vi "WPI_SonarSRF04DigitalGetRange.vi"(8 "error in (no error)":errorcluster, 10 "Range Units":T1, 11 "UltrasonicDevRef":T2={"DevStatus"={"status"=FALSE, "code"=0, "source"=""}, "Ping Channel"=enum."Invalid", "Echo Channel"=enum."Invalid", "CntIndex"=enum."Invalid"}) -> (0 "error out":errorcluster, 2 "Distance":dbl, 3 "UltrasonicDevRef":T2={"DevStatus"={"status"=FALSE, "code"=0, "source"=""}, "Ping Channel"=enum."Invalid", "Echo Channel"=enum."Invalid", "CntIndex"=enum."Invalid"})   [LabVIEW 2017]
doc: "Returns the distance, in inches or millimeters, between the ultrasonic sensor and the closest object in front of the sensor. The ultrasonic sensor measures this distance by emitting a ping and calculating the time it takes for the echo of the ping to return. If the ultrasonic sensor does not detect the echo of the ping in 50 ms or less, the VI times out and returns a <B>Distance</B> value of 0.\n\nThis software is licensed. Open the labview\\readme\\WPI Robotics Library Open Source License.txt file for more information."
uses:
  <vilib>/Rock Robotics/WPI/Ultrasonic/WPI_UltrasonicDeviceRef.ctl
  <vilib>/Rock Robotics/SystemInterfaces/DIO/FPGA_DIOChannel.ctl
  <vilib>/Rock Robotics/SystemInterfaces/Counter/FPGA_CounterCtrSystemIndex.ctl
  <vilib>/Rock Robotics/WPI/Ultrasonic/WPI_UltrasonicRangeUnits.ctl
  <instrlib>/Devantech SRF05/HAIOL/Devantech SRF05.lvclass
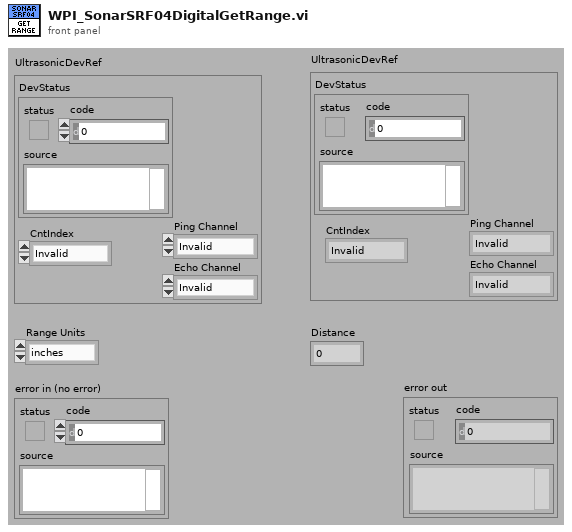
[diagram p1: front panel]
types:
  T1 = typedef "WPI_UltrasonicRangeUnits.ctl" = enum16{"inches", "mm"}
  T2 = typedef "WPI_UltrasonicDeviceRef.ctl" = cluster{"DevStatus":errorcluster, "Ping Channel":T3, "Echo Channel":T3, "CntIndex":T4}
  T3 = typedef "FPGA_DIOChannel.ctl" = enum8{"DIO 0", "DIO 1", "DIO 2", "DIO 3", "DIO 4", "DIO 5", "DIO 6", "DIO 7", "DIO 8", "DIO 9", "DIO MXP 0", "DIO MXP 1", "DIO MXP 2", "DIO MXP 3", "DIO MXP 4", "DIO MXP 5", "DIO MXP 6", "DIO MXP 7", "DIO MXP 8", "DIO MXP 9", "DIO MXP 10", "DIO MXP 11", "DIO MXP 12", "DIO MXP 13", "DIO MXP 14", "DIO MXP 15", "SPI Port CS1", "SPI Port CS2", "SPI Port CS3", "SPI Port MISO", "SPI Port MOSI", "Invalid"}
  T4 = typedef "FPGA_CounterCtrSystemIndex.ctl" = enum8{"Ctr 0", "Ctr 1", "Ctr 2", "Ctr 3", "Ctr 4", "Ctr 5", "Ctr 6", "Ctr 7", "Invalid"}
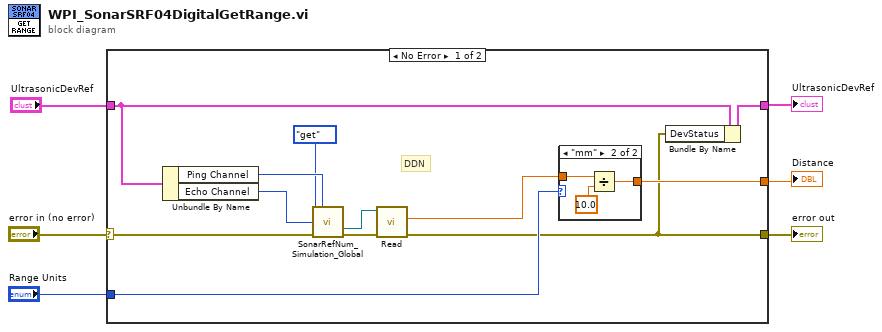
[diagram p0: block diagram]
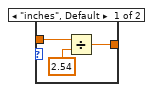
[diagram p2: hidden frame]
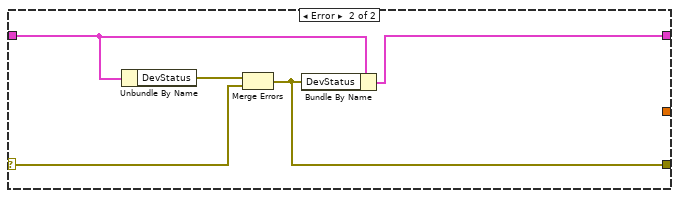
[diagram p3: hidden frame]
diagram:
  n1 = case shown="No Error" "error in (no error)" {
    selector: "error in (no error)" -> [w11 w26]
    tunnel: "UltrasonicDevRef" -> [w16 w29]
    tunnel: [w7 w28] -> w4
    tunnel: [w10 w25] -> w5
    tunnel: [w18 _] -> w6
    tunnel: "Range Units" -> [w17 _]
    frame No Error {
      # "DDN"
      n2 = Unbundle By Name(w16) -> ("Ping Channel"=w15:T3, "Echo Channel"=w8:T3)
      n3 = call <vilib>:"SonarRefNum_Simulation_Global.vi"("menu"=enum16{"set", "get", "delete"}."get", "Ping DIO Channel"=w15, "Echo DIO Channel"=w8, "error in (no error)"=w11) -> ("Devantech SRF05 Get"=w13:refnum<class "Devantech SRF05.lvclass">, "error out"=w12:errorcluster)  [unwired: 10 in]
      n4 = call-dynamic "Read.vi"("error in (no error)"=w12, "Devantech SRF05 in"=w13) -> ("error out"=w10:errorcluster, "Distance (cm)"=w9:dbl)  [unwired: 6 in, 2 out]
      n5 = case shown="\"mm\"" w17 {
        tunnel: w9 -> [w21 w24]
        tunnel: [w20 w23] -> w18
        frame "inches", Default {
          n6 = Divide(x=w21, y=2.54 ("uS to distance ratio")) -> (x/y=w20:dbl)
        }
        frame "mm" {
          n7 = Divide(x=w24, y=10.0 ("uS to distance ratio")) -> (x/y=w23:dbl)
        }
      }
      n8 = Bundle By Name(cluster=w16, "DevStatus"=w10) -> (w7:T2)
    }
    frame Error {
      n9 = Unbundle By Name(w29) -> ("DevStatus"=w27:errorcluster)
      n10 = Merge Errors(w27, w26) -> (w25:errorcluster)
      n11 = Bundle By Name(cluster=w29, "DevStatus"=w25) -> (w28:T2)
    }
  }
  "UltrasonicDevRef" <- w4
  "error out" <- w5
  "Distance" <- w6
